vi "plate_zero.vi"(8 "error in":errorcluster, 10 "DO array":bool[](array[boolean]), 11 "tasks":T2) -> (0 "error out":errorcluster, 3 "offsets":T1)   [LabVIEW 2013]
uses:
  <vilib>/DAQmx/write.llb/DAQmx Write (Digital 1D Bool NChan 1Samp 1Line).vi
  <vilib>/DAQmx/read.llb/DAQmx Read (Digital 1D Bool NChan 1Samp 1Line).vi
  <vilib>/DAQmx/read.llb/DAQmx Read (Counter DBL 1Chan 1Samp).vi
  <vilib>/DAQmx/configure/timing.llb/DAQmx Timing (Implicit).vi
  <vilib>/DAQmx/miscellaneous.llb/DAQmx Fill In Error Info.vi
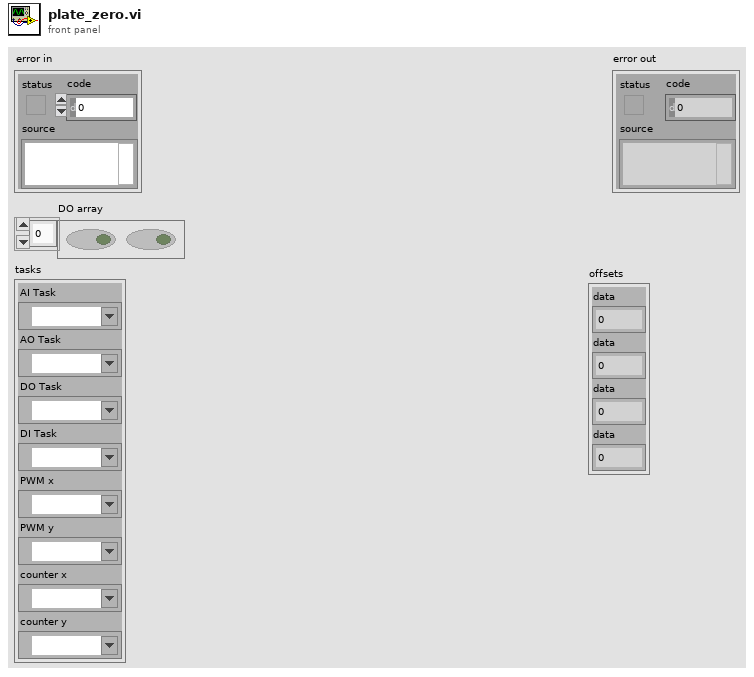
[diagram p1: front panel]
types:
  T1 = cluster{"data":dbl, "data":dbl, "data":dbl, "data":dbl}
  T2 = cluster{"AI Task":refnum<k21>, "AO Task":refnum<k21>, "DO Task":refnum<k21>, "DI Task":refnum<k21>, "PWM x":refnum<k21>, "PWM y":refnum<k21>, "counter x":refnum<k21>, "counter y":refnum<k21>}
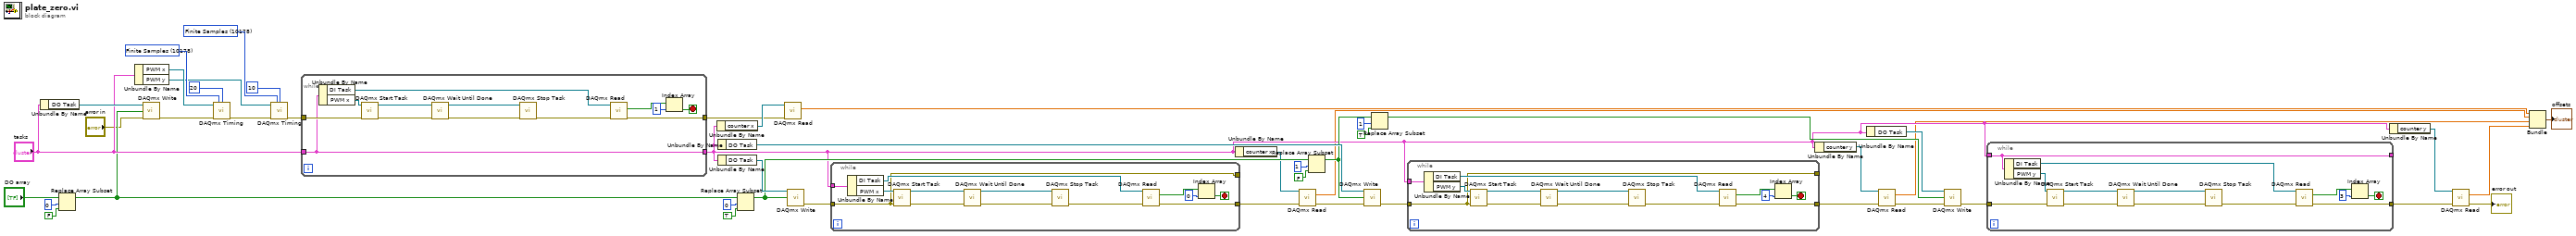
[diagram p0: block diagram]
diagram:
  w41 = 10178 items=["Finite Samples"=10178, "Continuous Samples"=10123, "Hardware Timed Single Point"=12522] ("sample mode")
  w43 = 10178 items=["Finite Samples"=10178, "Continuous Samples"=10123, "Hardware Timed Single Point"=12522] ("sample mode")
  n1 = Unbundle By Name("tasks") -> ("DO Task"=w45:refnum<k21>)
  n2 = Replace Array Subset(array="DO array", new element=FALSE ("new element/subarray"), index=0) -> (w26:bool[])
  n3 = Unbundle By Name("tasks") -> ("PWM x"=w44:refnum<k21>, "PWM y"=w39:refnum<k21>)
  n4 = call-poly <vilib>:"DAQmx Write.vi"("task/channels in"=w45, "data"=w26, "error in"="error in") -> ("error out"=w37:errorcluster)  [unwired: 10 in, 2 out]
  n5 = call-poly <vilib>:"DAQmx Timing.vi"("task/channels in"=w44, "sample mode"=w43, "samples per channel"=20, "error in"=w37) -> ("error out"=w38:errorcluster)  [unwired: 10 in, 1 out]
  n6 = call-poly <vilib>:"DAQmx Timing.vi"("task/channels in"=w39, "sample mode"=w41, "samples per channel"=10, "error in"=w38) -> ("error out"=w36:errorcluster)  [unwired: 10 in, 1 out]
  n7 = while {
    tunnel: w36 -> [w56]
    tunnel: "tasks" -> [w49]
    tunnel: [w50] -> w33
    tunnel: [w49] -> w9
    stop <- w58 stop-if-true
    n8 = Unbundle By Name(w49) -> ("DI Task"=w61:refnum<k21>, "PWM x"=w57:refnum<k21>)
    n9 = call <vilib>:"DAQmx Start Task.vi"("task/channels in"=w57, "error in"=w56) -> ("task out"=w54:refnum<k21>, "error out"=w55:errorcluster)  [unwired: 12 in]
    n10 = call <vilib>:"DAQmx Wait Until Done.vi"("task/channels in"=w54, "error in"=w55) -> ("task out"=w51:refnum<k21>, "error out"=w53:errorcluster)  [unwired: 12 in]
    n11 = call <vilib>:"DAQmx Stop Task.vi"("task/channels in"=w51, "error in"=w53) -> ("error out"=w52:errorcluster)  [unwired: 12 in, 1 out]
    n12 = call-poly <vilib>:"DAQmx Read.vi"("task/channels in"=w61, "error in"=w52) -> ("data"=w60:bool[], "error out"=w50:errorcluster)  [unwired: 11 in, 1 out]
    n13 = Index Array(array=w60, index=1) -> (element=w58:bool)
  }
  n14 = Unbundle By Name(w9) -> ("counter x"=w34:refnum<k21>)
  n15 = Unbundle By Name(w9) -> ("DO Task"=w27:refnum<k21>)
  n16 = Unbundle By Name(w9) -> ("DO Task"=w29:refnum<k21>)
  n17 = Replace Array Subset(array=w26, new element=TRUE ("new element/subarray"), index=0) -> (w25:bool[])
  n18 = call-poly <vilib>:"DAQmx Read.vi"("task/channels in"=w34, "error in"=w33) -> ("data"=w7:dbl)  [unwired: 11 in, 2 out]
  n19 = call-poly <vilib>:"DAQmx Write.vi"("task/channels in"=w29, "data"=w25) -> ("error out"=w32:errorcluster)  [unwired: 11 in, 2 out]
  n20 = while {
    tunnel: [w62] -> _
    tunnel: w9 -> [w74]
    tunnel: [w63] -> w22
    tunnel: w32 -> [w62]
    stop <- w70 stop-if-true
    n21 = Unbundle By Name(w74) -> ("DI Task"=w73:refnum<k21>, "PWM x"=w69:refnum<k21>)
    n22 = call <vilib>:"DAQmx Start Task.vi"("task/channels in"=w69, "error in"=w62) -> ("task out"=w67:refnum<k21>, "error out"=w68:errorcluster)  [unwired: 12 in]
    n23 = call <vilib>:"DAQmx Wait Until Done.vi"("task/channels in"=w67, "error in"=w68) -> ("task out"=w64:refnum<k21>, "error out"=w66:errorcluster)  [unwired: 12 in]
    n24 = call <vilib>:"DAQmx Stop Task.vi"("task/channels in"=w64, "error in"=w66) -> ("error out"=w65:errorcluster)  [unwired: 12 in, 1 out]
    n25 = call-poly <vilib>:"DAQmx Read.vi"("task/channels in"=w73, "error in"=w65) -> ("data"=w72:bool[], "error out"=w63:errorcluster)  [unwired: 11 in, 1 out]
    n26 = Index Array(array=w72, index=0) -> (element=w70:bool)
  }
  n27 = Unbundle By Name(w9) -> ("counter x"=w20:refnum<k21>)
  n28 = call-poly <vilib>:"DAQmx Read.vi"("task/channels in"=w20, "error in"=w22) -> ("data"=w6:dbl, "error out"=w21:errorcluster)  [unwired: 11 in, 1 out]
  n29 = Replace Array Subset(array=w25, new element=FALSE ("new element/subarray"), index=1) -> (w14:bool[])
  n30 = call-poly <vilib>:"DAQmx Write.vi"("task/channels in"=w27, "data"=w14, "error in"=w21) -> ("error out"=w28:errorcluster)  [unwired: 10 in, 2 out]
  n31 = Replace Array Subset(array=w14, new element=TRUE ("new element/subarray"), index=1) -> (w11:bool[])
  n32 = while {
    tunnel: [w75] -> _
    tunnel: w9 -> [w87]
    tunnel: [w76] -> w19
    tunnel: w28 -> [w75]
    stop <- w83 stop-if-true
    n33 = Unbundle By Name(w87) -> ("DI Task"=w86:refnum<k21>, "PWM y"=w82:refnum<k21>)
    n34 = call <vilib>:"DAQmx Start Task.vi"("task/channels in"=w82, "error in"=w75) -> ("task out"=w80:refnum<k21>, "error out"=w81:errorcluster)  [unwired: 12 in]
    n35 = call <vilib>:"DAQmx Wait Until Done.vi"("task/channels in"=w80, "error in"=w81) -> ("task out"=w77:refnum<k21>, "error out"=w79:errorcluster)  [unwired: 12 in]
    n36 = call <vilib>:"DAQmx Stop Task.vi"("task/channels in"=w77, "error in"=w79) -> ("error out"=w78:errorcluster)  [unwired: 12 in, 1 out]
    n37 = call-poly <vilib>:"DAQmx Read.vi"("task/channels in"=w86, "error in"=w78) -> ("data"=w85:bool[], "error out"=w76:errorcluster)  [unwired: 11 in, 1 out]
    n38 = Index Array(array=w85, index=4) -> (element=w83:bool)
  }
  n39 = Unbundle By Name(w9) -> ("counter y"=w18:refnum<k21>)
  n40 = Unbundle By Name(w9) -> ("DO Task"=w16:refnum<k21>)
  n41 = call-poly <vilib>:"DAQmx Read.vi"("task/channels in"=w18, "error in"=w19) -> ("data"=w5:dbl, "error out"=w17:errorcluster)  [unwired: 11 in, 1 out]
  n42 = call-poly <vilib>:"DAQmx Write.vi"("task/channels in"=w16, "data"=w11, "error in"=w17) -> ("error out"=w15:errorcluster)  [unwired: 10 in, 2 out]
  n43 = while {
    tunnel: w15 -> [w89]
    tunnel: [w88] -> _
    tunnel: [w90] -> w10
    tunnel: w9 -> [w88]
    stop <- w97 stop-if-true
    n44 = Unbundle By Name(w88) -> ("DI Task"=w100:refnum<k21>, "PWM y"=w96:refnum<k21>)
    n45 = call <vilib>:"DAQmx Start Task.vi"("task/channels in"=w96, "error in"=w89) -> ("task out"=w94:refnum<k21>, "error out"=w95:errorcluster)  [unwired: 12 in]
    n46 = call <vilib>:"DAQmx Wait Until Done.vi"("task/channels in"=w94, "error in"=w95) -> ("task out"=w91:refnum<k21>, "error out"=w93:errorcluster)  [unwired: 12 in]
    n47 = call <vilib>:"DAQmx Stop Task.vi"("task/channels in"=w91, "error in"=w93) -> ("error out"=w92:errorcluster)  [unwired: 12 in, 1 out]
    n48 = call-poly <vilib>:"DAQmx Read.vi"("task/channels in"=w100, "error in"=w92) -> ("data"=w99:bool[], "error out"=w90:errorcluster)  [unwired: 11 in, 1 out]
    n49 = Index Array(array=w99, index=3) -> (element=w97:bool)
  }
  n50 = Unbundle By Name(w9) -> ("counter y"=w8:refnum<k21>)
  n51 = call-poly <vilib>:"DAQmx Read.vi"("task/channels in"=w8, "error in"=w10) -> ("data"=w4:dbl, "error out"=→"error out":errorcluster)  [unwired: 11 in, 1 out]
  n52 = Bundle("data"=w7, "data"=w6, "data"=w5, "data"=w4) -> (→"offsets":T1)  [unwired: 1 in]
